vi "Forward Kinematics (Trajectory).vi"(8 "error in (no error)":errorcluster, 10 "joint position trajectory":dbl[][](array[numeric]), 11 "serial arm in":refnum<class "NI_Robotics_Serial Robot Arm.lvclass">) -> (0 "error out":errorcluster, 2 "end effector transforms":dbl[][][](array[numeric]), 3 "serial arm out":refnum<class "NI_Robotics_Serial Robot Arm.lvclass">)   [LabVIEW 2017, in "NI_Kinematics.lvlib"]
doc: "Returns a homogenous transform or transforms that represents the position of a robotic arm end effector given the joint angles of the arm. Wire data to the <B>joint positions</B> input to determine the polymorphic instance to use or manually select the instance.\n\n<B>.m file:</B> fkine"
uses:
  <vilib>/robotics/Kinematics/NI_Kinematics.lvlib
  <vilib>/robotics/Kinematics/Robot/NI_Robotics_Serial Robot Arm.lvclass
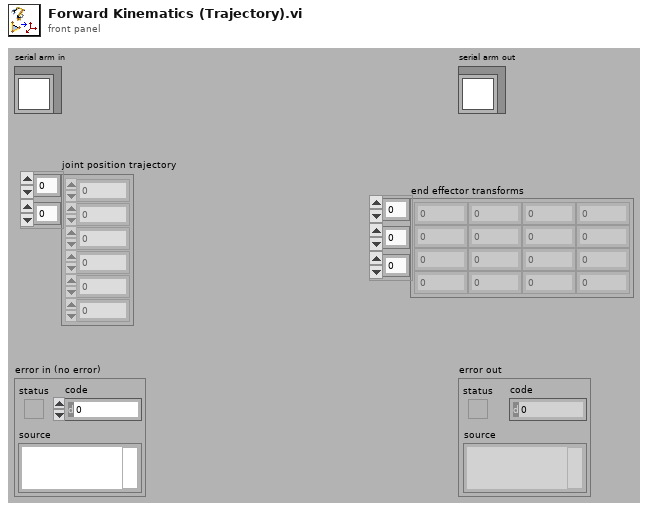
[diagram p1: front panel]
types:
  T1 = typedef "NI_Matrix.lvlib/RealMatrix.ctl" = dbl[][]
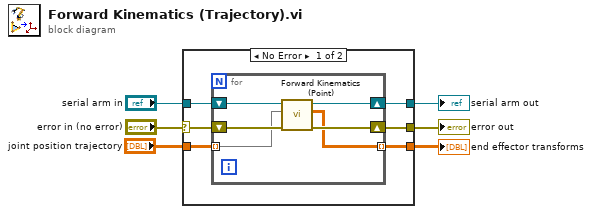
[diagram p0: block diagram]
diagram:
  n1 = case shown="No Error" "error in (no error)" {
    selector: "error in (no error)" -> [w12 w20]
    tunnel: [w8 w20] -> w5
    tunnel: [w9 w19] -> w3
    tunnel: "serial arm in" -> [w10 w19]
    tunnel: "joint position trajectory" -> [w11 _]
    tunnel: [w7 _] -> w1
    frame No Error {
      n2 = for {
        shift-right: [w15] -> w8
        shift-left: w12 -> [w16]
        tunnel: w11 -> [w14] mode=indexing
        shift-right: [w17] -> w9
        shift-left: w10 -> [w18]
        tunnel: [w13] -> w7 mode=indexing
        n3 = call <vilib>:"Forward Kinematics (Point).vi"("error in (no error)"=w16, "joint positions"=w14, "serial arm in"=w18) -> ("error out"=w15:errorcluster, "end effector transform"=w13:T1, "serial arm out"=w17:refnum<class "NI_Robotics_Serial Robot Arm.lvclass">)  [unwired: 6 out]
      }
    }
    frame Error {
    }
  }
  "error out" <- w5
  "serial arm out" <- w3
  "end effector transforms" <- w1
